vi "Detect Items Being Dragged.vi"(7 "ListBox":refnum<vi>, 8 "error in (no error)":errorcluster, 10 "LB Filenames":string[](array[string]), 11 "Data":T1(array[cluster])) -> (0 "error out":errorcluster, 2 "Colors":u32[](array[colorbox]), 3 "Items Dragged":string[](array[string]))   [LabVIEW 2011]
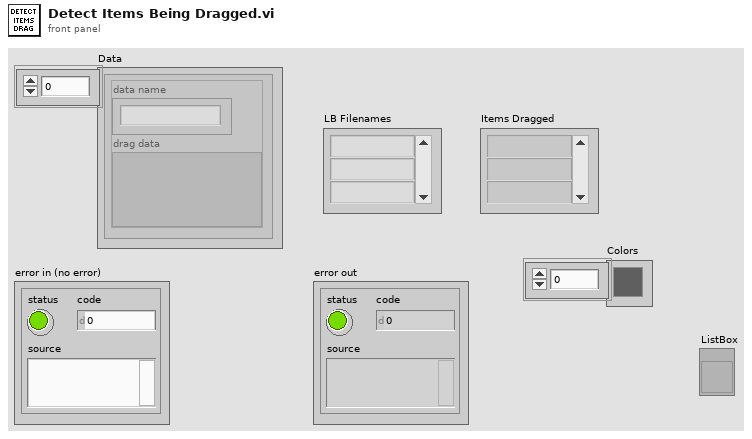
[diagram p1: front panel]
types:
  T1 = cluster{"data name":string, "drag data":variant}[]
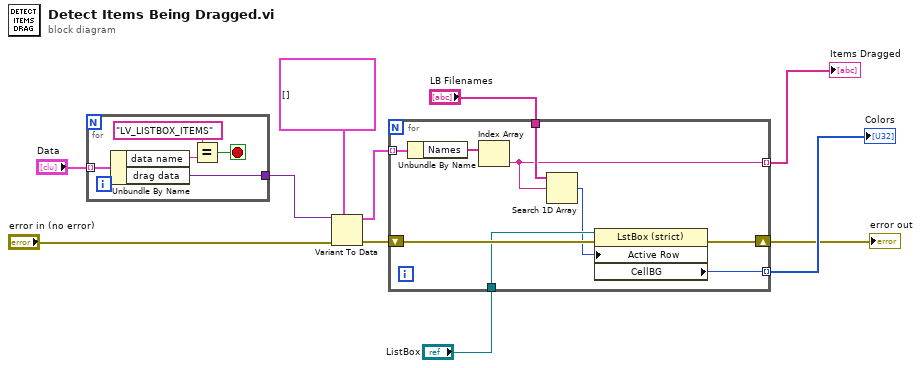
[diagram p0: block diagram]
diagram:
  n1 = for {
    tunnel: "Data" -> [w16] mode=indexing
    tunnel: [w13] -> w11
    stop <- w12 stop-if-true
    n2 = Unbundle By Name(w16) -> ("data name"=w15:string, "drag data"=w13:variant)
    n3 = Equal?(x="LV_LISTBOX_ITEMS", y=w15) -> (x = y?=w12:bool)
  }
  n4 = Variant To Data(error in="error in (no error)", type=cluster{"Names":string[], i32}[] [], Variant=w11) -> (data=w7:cluster{"Names":string[], i32}[], error out=w4:errorcluster)
  n5 = for {
    tunnel: w7 -> [w25] mode=indexing
    tunnel: [w22] -> w6 mode=indexing
    tunnel: "LB Filenames" -> [w23]
    shift-right: [w18] -> w1
    shift-left: w4 -> [w21]
    tunnel: "ListBox" -> [w20]
    tunnel: [w17] -> w2 mode=indexing
    n6 = Unbundle By Name(w25) -> ("Names"=w24:string[])
    n7 = Index Array(array=w24) -> (element=w22:string)  [unwired: 1 in]
    n8 = Search 1D Array(1D array=w23, element=w22) -> (index of element=w19:i32)  [unwired: 1 in]
    n9 = property class="LstBox (strict)"(reference=w20, error in=w21, "Active Row"=w19) -> (error out=w18:errorcluster, "CellBG"=w17:u32)  [unwired: 1 out]
  }
  "error out" <- w1
  "Colors" <- w2
  "Items Dragged" <- w6
